vi "Enqueue Message (Single).vi"(6 "Priority Message? (F)":bool, 8 "error in (no error)":errorcluster, 9 "Message Data":variant, 10 "Message":string, 11 "Message Queue":refnum<queue>) -> (0 "error out":errorcluster, 3 "dup Message Queue":refnum<queue>)   [LabVIEW 2013, in "Message Queue.lvlib"]
doc: "For a regular message, enqueue the message. For a priority message, enqueue it at the front of the queue."
uses:
  Message Queue.lvlib
  Message Cluster.ctl
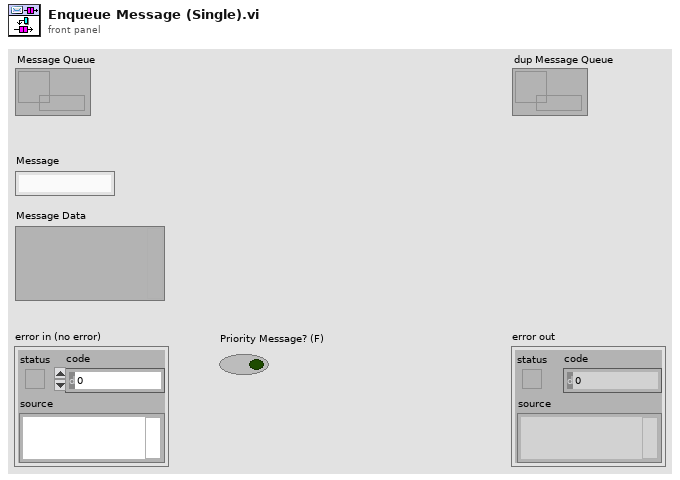
[diagram p1: front panel]
types:
  T1 = typedef "Message Queue.lvlib/Message Cluster.ctl" = cluster{"Message":string, "Message Data":variant}
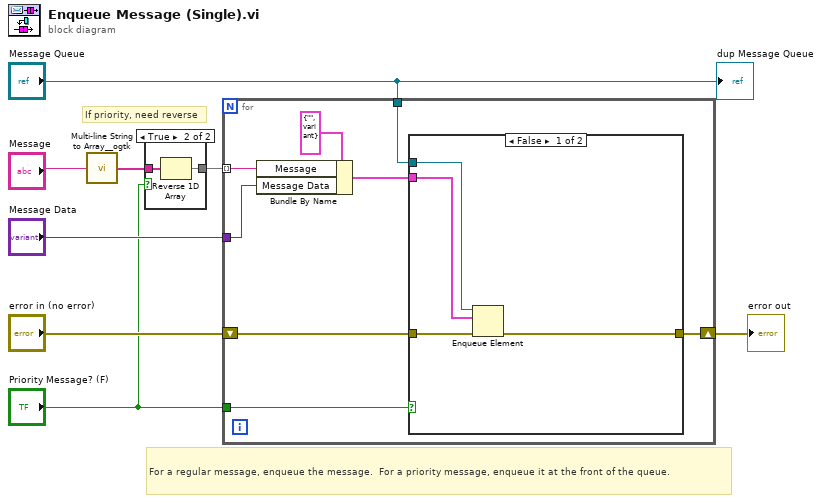
[diagram p0: block diagram]
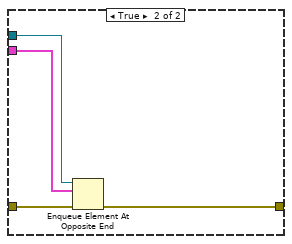
[diagram p3: hidden frame]
diagram:
  # "If priority, need reverse"
  # "For a regular message, enqueue the message.  For a priority message, enqueue it at the front of the queue."
  n1 = call <userlib>:"Multi-line String to Array__ogtk.vi"("string"="Message") -> ("lines"=w3:string[])
  n2 = case shown="True" "Priority Message? (F)" {
    tunnel: w3 -> [w9 w11]
    tunnel: [w9 w10] -> w2
    frame False {
    }
    frame True {
      n3 = Reverse 1D Array(array=w11) -> (reversed array=w10:string[])
    }
  }
  n4 = for {
    tunnel: "Message Data" -> [w18]
    tunnel: "Priority Message? (F)" -> [w17]
    tunnel: "Message Queue" -> [w14]
    shift-right: [w15] -> w5
    shift-left: "error in (no error)" -> [w16]
    tunnel: w2 -> [w12] mode=indexing
    n5 = Bundle By Name(cluster=T1 {"Message"="", "Message Data"=variant} ("Message Cluster"), "Message"=w12, "Message Data"=w18) -> (w13:T1)
    n6 = case shown="False" w17 {
      tunnel: w16 -> [w23 w27]
      tunnel: [w22 w26] -> w15
      tunnel: w14 -> [w21 w25]
      tunnel: w13 -> [w20 w24]
      frame False {
        n7 = Enqueue Element(queue=w21, element=w20, error in (no error)=w23) -> (error out=w22:errorcluster)  [unwired: 1 in, 2 out]
      }
      frame True {
        n8 = Enqueue Element At Opposite End(queue=w25, element=w24, error in (no error)=w27) -> (error out=w26:errorcluster)  [unwired: 1 in, 2 out]
      }
    }
  }
  "error out" <- w5
  "dup Message Queue" <- "Message Queue"
